vi "FPGA_LASER_4SETUP_Feb19_2016.vi"() -> ()   [LabVIEW 2015]
uses:
  <vilib>/rvi/Emulation/niFpgaGetClockAttributes.vi
  <vilib>/rvi/Emulation/niFpgaSctlEmulationGetInTimedLoop.vi
  <vilib>/rvi/Emulation/niFpgaEmulationReportErrorSimple.vi
  <vilib>/rvi/eio/common/nirviEmuTemplateMethod_errors.vi
  <vilib>/rvi/interface/RandomDataEmulation/niFpgaRandomDataHandleErrors.vi
  <vilib>/rvi/Emulation/niFpgaCriticalErrorInLSC.vi
  <vilib>/eio/EIONode/EIONode.xnode
  <vilib>/rvi/DataTransferAndStorage/Container/XNode/niFpgaContainer.xnode
  <vilib>/rvi/interface/RandomDataEmulation/nirviRandomDataFpgaReadWriteTemplate.vi
panel:
  out "Tick Count(Ticks) J5":u32 caption="Tick Count(Ticks)"
  out "Tick Count(Ticks) J8":u32 caption="Tick Count(Ticks)"
  out "Tick Count(Ticks) J4":u32 caption="Tick Count(Ticks)"
  out "Tick Count(Ticks) J1":u32 caption="Tick Count(Ticks)"
  in  "stop LED illumination J8":bool
  in  "Low Period (ticks) J8":u32=40000000
  in  "High Period (ticks) J8":u32=40000000
  in  "Apply J8":bool
  in  "Output Enable J8":bool
  in  "FPGA Stop J8":bool
  in  "Half-clock time J8":u32=10
  out "ConnectorA/DIO0 J8":bool=TRUE
  out "Frame Count J8":i16=5
  in  "IRQ Bit (0-31) J8":u8
  in  "Wait Until IRQ Cleared? J8":bool
  out "Timed Out? J8":bool
  out "ConnectorA/AI0 J8":u16=44020
  out "ConnectorA/DIO1 J8":bool
  in  "double number of samples to take per frame J8":u16=1540
  in  "Half-clocks between frames J8":u16=1600
  in  "ConnectorA/AO1 J8":u16
  in  "stop LED illumination J4":bool
  in  "Low Period (ticks) J4":u32=40000000
  in  "High Period (ticks) J4":u32=40000000
  in  "Apply J4":bool
  in  "Output Enable J4":bool
  in  "FPGA Stop J4":bool
  in  "Half-clock time J4":u32=10
  out "ConnectorB/DIO0 J4":bool=TRUE
  out "Frame Count J4":i16=5
  in  "IRQ Bit (0-31) J4":u8
  in  "Wait Until IRQ Cleared? J4":bool
  out "Timed Out? J4":bool
  out "ConnectorB/AI0 J4":u16=44020
  out "ConnectorB/DIO1 J4":bool
  in  "double number of samples to take per frame J4":u16=1540
  in  "Half-clocks between frames J4":u16=1600
  in  "ConnectorB/AO1 J4":u16
  in  "stop LED illumination J5":bool
  in  "Low Period (ticks) J5":u32=40000000
  in  "High Period (ticks) J5":u32=40000000
  in  "Apply J5":bool
  in  "Output Enable J5":bool
  in  "FPGA Stop J5":bool
  in  "Half-clock time J5":u32=10
  out "ConnectorA/DIO0 J5":bool=TRUE
  out "Frame Count J5":i16=5
  in  "IRQ Bit (0-31) J5":u8
  in  "Wait Until IRQ Cleared? J5":bool
  out "Timed Out? J5":bool
  out "ConnectorA/AI0 J5":u16=44020
  out "ConnectorA/DIO1 J5":bool
  in  "double number of samples to take per frame J5":u16=1540
  in  "Half-clocks between frames J5":u16=1600
  in  "ConnectorA/AO0 J5":u16
  in  "stop LED illumination J1":bool
  in  "Low Period (ticks) J1":u32=40000000
  in  "High Period (ticks) J1":u32=40000000
  in  "Apply J1":bool
  in  "Output Enable J1":bool
  in  "FPGA Stop J1":bool
  in  "Half-clock time J1":u32=10
  out "ConnectorB/DIO0, J1":bool=TRUE
  out "Frame Count J1":i16=5
  in  "IRQ Bit (0-31) J1":u8
  in  "Wait Until IRQ Cleared? J1":bool
  out "Timed Out? J1":bool
  out "ConnectorB/AI0 J1":u16=44020
  out "ConnectorB/DIO1 J1":bool
  in  "double number of samples to take per frame J1":u16=1540
  in  "Half-clocks between frames J1":u16=1600
  in  "ConnectorB/AO0 J1":u16
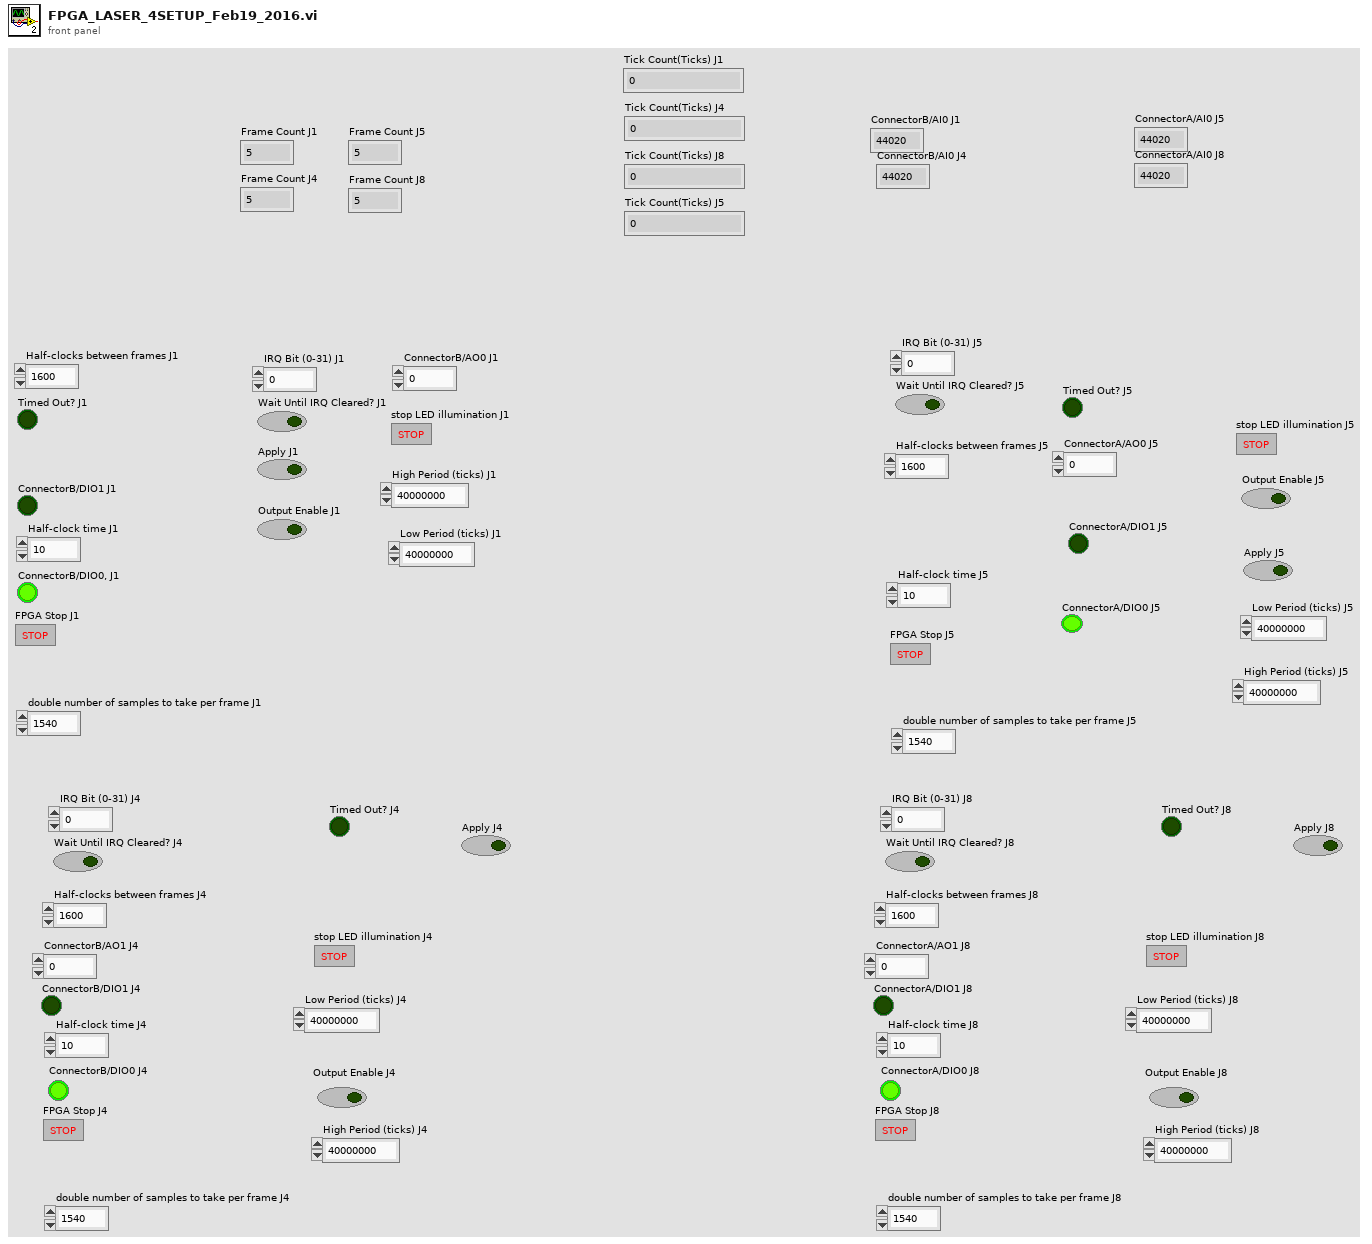
[diagram p1: front panel]
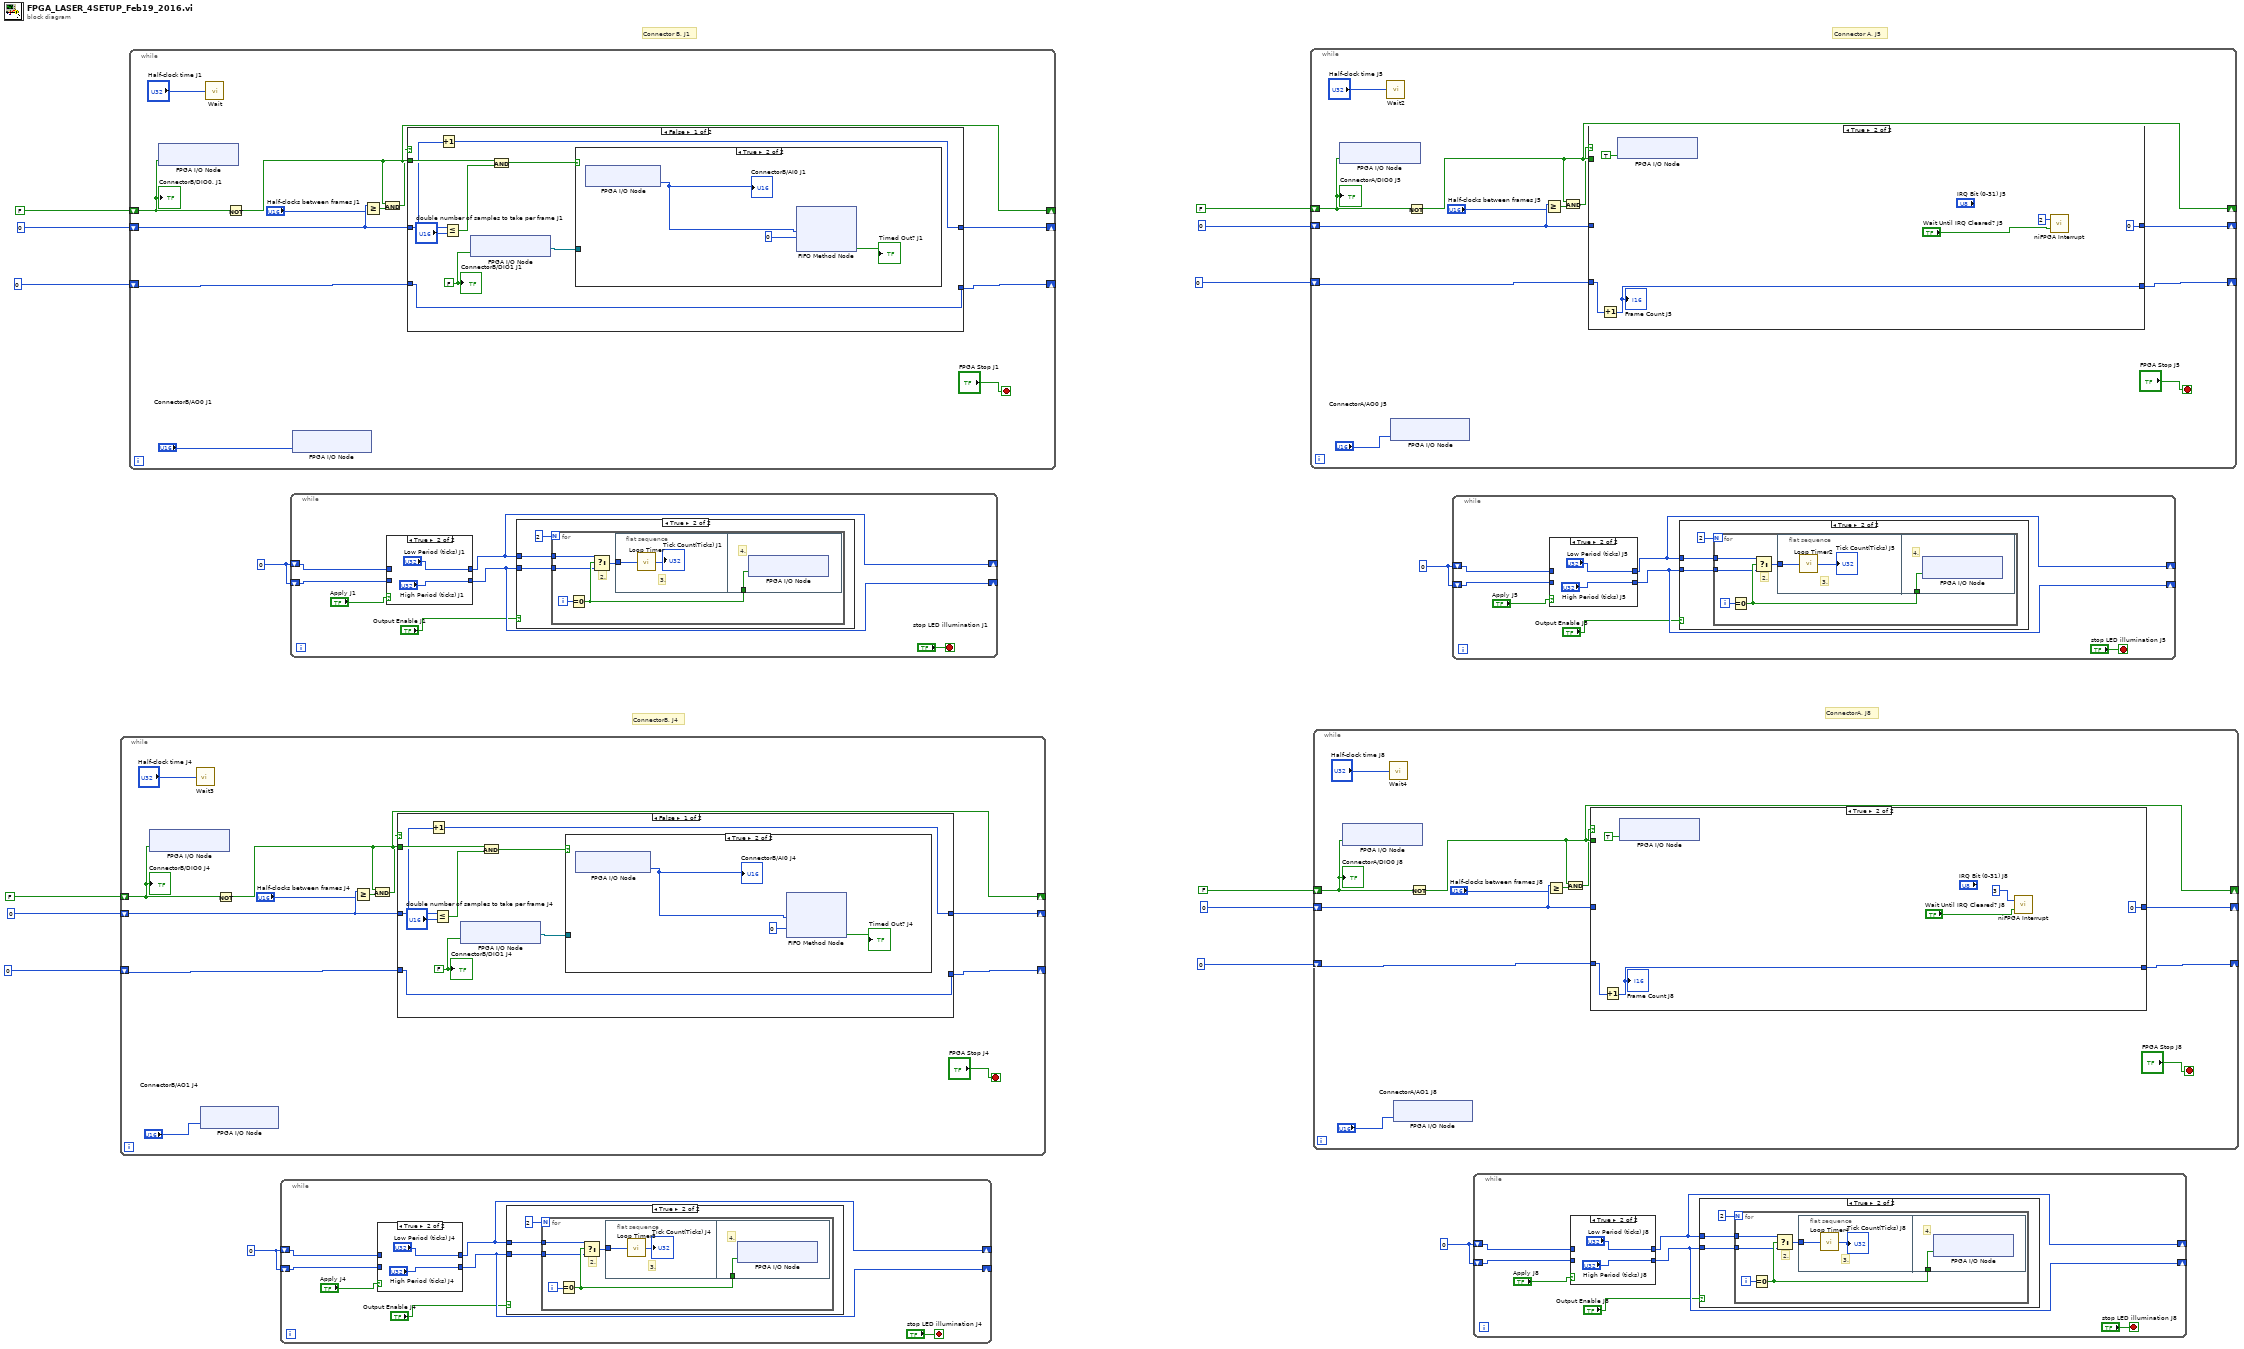
[diagram p0: block diagram]
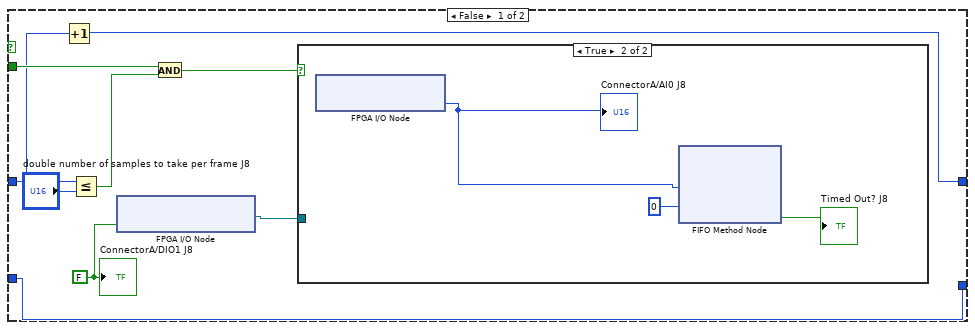
[diagram p4: hidden frame]
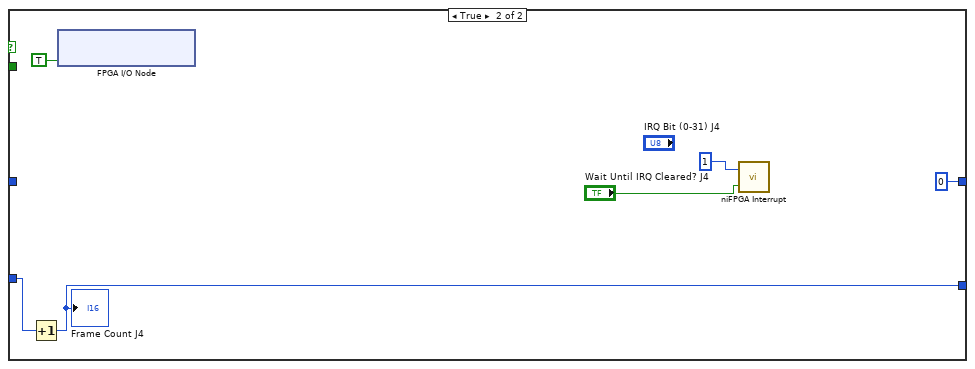
[diagram p9: hidden frame]
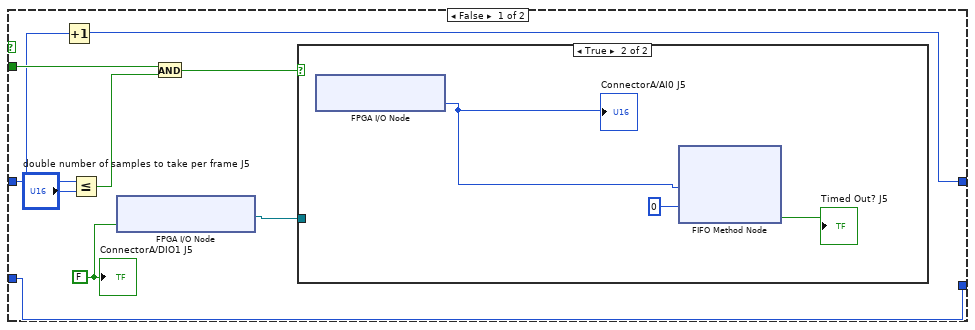
[diagram p12: hidden frame]
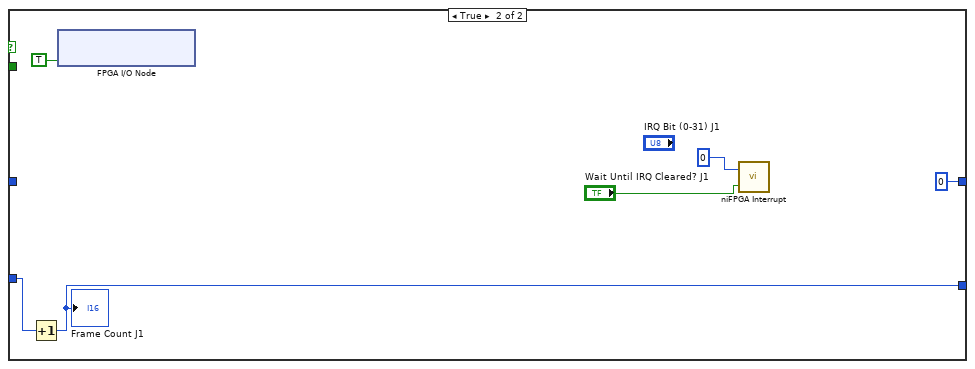
[diagram p17: hidden frame]
diagram:
  w1 = u32 0 ("High Period")
  w5 = u32 0 ("High Period")
  w9 = u32 0 ("High Period")
  w13 = u32 0 ("High Period")
  # "ConnectorA, J8"
  # "ConnectorB, J4"
  # "Connector A, J5"
  # "Connector B, J1"
  n1 = while {
    shift-right: [w27] -> _
    shift-left: FALSE ("ConnectorB/DIO0") -> [w28]
    shift-right: [w24] -> _
    shift-left: u16 0 -> [w26]
    shift-right: [w22] -> _
    shift-left: i16 0 -> [w23]
    stop <- "FPGA Stop J4" stop-if-true
    n2 = xnode "FPGA I/O Node"("ConnectorB/DIO2"=w28) -> ()  [unwired: 1 in, 1 out]
    n3 = call "Wait3"("Count(uSec)"="Half-clock time J4") -> ()  [unwired: 1 out]
    n4 = xnode "FPGA I/O Node"("ConnectorB/AO1"="ConnectorB/AO1 J4") -> ()  [unwired: 1 in, 1 out]
    n5 = Not(x=w28) -> (.not. x?=w27:bool)
    n6 = Greater Or Equal?(x=w26, y="Half-clocks between frames J4") -> (x >= y?=w20:bool)
    n7 = And(x=w27, y=w20) -> (x .and. y?=w18:bool)
    n8 = case shown="False" w18 {
      tunnel: w26 -> [w32 _]
      tunnel: [w30 u16 0] -> w24
      tunnel: w27 -> [w36 _]
      tunnel: w23 -> [w31 w44]
      tunnel: [w31 w43] -> w22
      frame False {
        w37 = FALSE ("ConnectorB/DIO1")
        n9 = Increment(x=w32) -> (x+1=w30:u16)
        n10 = Less Or Equal?(x=w32, y="double number of samples to take per frame J4") -> (x <= y?=w34:bool)
        n11 = xnode "FPGA I/O Node"("ConnectorB/DIO3"=w37) -> ("FPGA I/O Out"=w33:refnum<k21>)  [unwired: 1 in]
        n12 = And(x=w36, y=w34) -> (x .and. y?=w35:bool)
        n13 = case shown="True" w35 {
          tunnel: w33 -> [_ _]
          frame False {
          }
          frame True {
            n14 = xnode "FPGA I/O Node"() -> ("ConnectorB/AI1"=w40:u16)  [unwired: 1 in, 1 out]
            "ConnectorB/AI0 J4" <- w40
            n15 = xnode ("FIFO Method Node")("Element"=w40, "Timeout"=0) -> ("Timed Out?"=→"Timed Out? J4":bool)  [unwired: 1 in, 1 out]
          }
        }
        "ConnectorB/DIO1 J4" <- w37
      }
      frame True {
        n16 = Increment(x=w44) -> (x+1=w43:i16)
        "Frame Count J4" <- w43
        n17 = xnode "FPGA I/O Node"("ConnectorB/DIO3"=TRUE ("ConnectorB/DIO1")) -> ()  [unwired: 1 in, 1 out]
        n18 = call <vilib>:"niFPGA Interrupt.vi"("Wait Until Cleared (F)"="Wait Until IRQ Cleared? J4", "IRQ Number (0)"=u8 1) -> ()  [unwired: 1 in]
      }
    }
    "ConnectorB/DIO0 J4" <- w28
  }
  n19 = while {
    shift-right: [w57] -> _
    shift-left: FALSE ("ConnectorB/DIO0") -> [w58]
    shift-right: [w54] -> _
    shift-left: u16 0 -> [w56]
    shift-right: [w52] -> _
    shift-left: i16 0 -> [w53]
    stop <- "FPGA Stop J1" stop-if-true
    n20 = xnode "FPGA I/O Node"("ConnectorB/DIO0"=w58) -> ()  [unwired: 1 in, 1 out]
    n21 = call "Wait"("Count(uSec)"="Half-clock time J1") -> ()  [unwired: 1 out]
    n22 = Not(x=w58) -> (.not. x?=w57:bool)
    n23 = xnode "FPGA I/O Node"("ConnectorB/AO0"="ConnectorB/AO0 J1") -> ()  [unwired: 1 in, 1 out]
    n24 = Greater Or Equal?(x=w56, y="Half-clocks between frames J1") -> (x >= y?=w50:bool)
    n25 = And(x=w57, y=w50) -> (x .and. y?=w48:bool)
    n26 = case shown="False" w48 {
      tunnel: w56 -> [w62 _]
      tunnel: [w60 u16 0] -> w54
      tunnel: w57 -> [w66 _]
      tunnel: w53 -> [w61 w74]
      tunnel: [w61 w73] -> w52
      frame False {
        w67 = FALSE ("ConnectorB/DIO1")
        n27 = Increment(x=w62) -> (x+1=w60:u16)
        n28 = Less Or Equal?(x=w62, y="double number of samples to take per frame J1") -> (x <= y?=w64:bool)
        n29 = xnode "FPGA I/O Node"("ConnectorB/DIO1"=w67) -> ("FPGA I/O Out"=w63:refnum<k21>)  [unwired: 1 in]
        n30 = And(x=w66, y=w64) -> (x .and. y?=w65:bool)
        n31 = case shown="True" w65 {
          tunnel: w63 -> [_ _]
          frame False {
          }
          frame True {
            n32 = xnode "FPGA I/O Node"() -> ("ConnectorB/AI0"=w70:u16)  [unwired: 1 in, 1 out]
            "ConnectorB/AI0 J1" <- w70
            n33 = xnode ("FIFO Method Node")("Element"=w70, "Timeout"=0) -> ("Timed Out?"=→"Timed Out? J1":bool)  [unwired: 1 in, 1 out]
          }
        }
        "ConnectorB/DIO1 J1" <- w67
      }
      frame True {
        n34 = Increment(x=w74) -> (x+1=w73:i16)
        "Frame Count J1" <- w73
        n35 = xnode "FPGA I/O Node"("ConnectorB/DIO1"=TRUE) -> ()  [unwired: 1 in, 1 out]
        n36 = call <vilib>:"niFPGA Interrupt.vi"("Wait Until Cleared (F)"="Wait Until IRQ Cleared? J1", "IRQ Number (0)"=u8 0) -> ()  [unwired: 1 in]
      }
    }
    "ConnectorB/DIO0, J1" <- w58
  }
  n37 = while {
    shift-right: [w78] -> _
    shift-left: w5 -> [w82]
    shift-right: [w79] -> _
    shift-left: w5 -> [w81]
    stop <- "stop LED illumination J4" stop-if-true
    n38 = case shown="True" "Apply J4" {
      tunnel: [w96 "Low Period (ticks) J4"] -> w78
      tunnel: [w95 "High Period (ticks) J4"] -> w79
      tunnel: w82 -> [w96 _]
      tunnel: w81 -> [w95 _]
      frame False {
      }
      frame True {
      }
    }
    n39 = case shown="True" "Output Enable J4" {
      tunnel: w78 -> [_ w85]
      tunnel: w79 -> [_ w84]
      frame False {
      }
      frame True {
        n40 = for {
          N: 2 -> [_]
          tunnel: w85 -> [w88]
          tunnel: w84 -> [w87]
          i -> [w90]
          # "2."
          n41 = Equal To 0?(x=w90) -> (x = 0?=w89:bool)
          n42 = Select(t=w88, s=w89, f=w87) -> (s? t:f=w91:u32)
          n43 = flat-sequence {
            tunnel: w91 -> [w93]
            tunnel: w89 -> [w94]
            frame #0 {
              # "3."
              n44 = call "Loop Timer3"("Count(Ticks)"=w93) -> ("Tick Count(Ticks)"=→"Tick Count(Ticks) J4":u32)
            }
            frame #1 {
              # "4."
              n45 = xnode "FPGA I/O Node"("ConnectorB/DIO9"=w94) -> ()  [unwired: 1 in, 1 out]
            }
          }
        }
      }
    }
  }
  n46 = while {
    shift-right: [w100] -> _
    shift-left: w13 -> [w104]
    shift-right: [w101] -> _
    shift-left: w13 -> [w103]
    stop <- "stop LED illumination J1" stop-if-true
    n47 = case shown="True" "Apply J1" {
      tunnel: [w118 "Low Period (ticks) J1"] -> w100
      tunnel: [w117 "High Period (ticks) J1"] -> w101
      tunnel: w104 -> [w118 _]
      tunnel: w103 -> [w117 _]
      frame False {
      }
      frame True {
      }
    }
    n48 = case shown="True" "Output Enable J1" {
      tunnel: w100 -> [_ w107]
      tunnel: w101 -> [_ w106]
      frame False {
      }
      frame True {
        n49 = for {
          N: 2 -> [_]
          tunnel: w107 -> [w110]
          tunnel: w106 -> [w109]
          i -> [w112]
          # "2."
          n50 = Equal To 0?(x=w112) -> (x = 0?=w111:bool)
          n51 = Select(t=w110, s=w111, f=w109) -> (s? t:f=w113:u32)
          n52 = flat-sequence {
            tunnel: w113 -> [w115]
            tunnel: w111 -> [w116]
            frame #0 {
              # "3."
              n53 = call "Loop Timer"("Count(Ticks)"=w115) -> ("Tick Count(Ticks)"=→"Tick Count(Ticks) J1":u32)
            }
            frame #1 {
              # "4."
              n54 = xnode "FPGA I/O Node"("ConnectorB/DIO8"=w116) -> ()  [unwired: 1 in, 1 out]
            }
          }
        }
      }
    }
  }
  n55 = while {
    shift-right: [w131] -> _
    shift-left: FALSE ("ConnectorB/DIO0") -> [w132]
    shift-right: [w128] -> _
    shift-left: u16 0 -> [w130]
    shift-right: [w126] -> _
    shift-left: i16 0 -> [w127]
    stop <- "FPGA Stop J5" stop-if-true
    n56 = xnode "FPGA I/O Node"("ConnectorA/DIO0"=w132) -> ()  [unwired: 1 in, 1 out]
    n57 = call "Wait2"("Count(uSec)"="Half-clock time J5") -> ()  [unwired: 1 out]
    n58 = xnode "FPGA I/O Node"("ConnectorA/AO0"="ConnectorA/AO0 J5") -> ()  [unwired: 1 in, 1 out]
    n59 = Not(x=w132) -> (.not. x?=w131:bool)
    n60 = Greater Or Equal?(x=w130, y="Half-clocks between frames J5") -> (x >= y?=w124:bool)
    n61 = And(x=w131, y=w124) -> (x .and. y?=w122:bool)
    n62 = case shown="True" w122 {
      tunnel: w130 -> [w136 _]
      tunnel: [w134 u16 0] -> w128
      tunnel: w131 -> [w140 _]
      tunnel: w127 -> [w135 w148]
      tunnel: [w135 w147] -> w126
      frame False {
        w141 = FALSE ("ConnectorB/DIO1")
        n63 = Increment(x=w136) -> (x+1=w134:u16)
        n64 = Less Or Equal?(x=w136, y="double number of samples to take per frame J5") -> (x <= y?=w138:bool)
        n65 = xnode "FPGA I/O Node"("ConnectorA/DIO1"=w141) -> ("FPGA I/O Out"=w137:refnum<k21>)  [unwired: 1 in]
        n66 = And(x=w140, y=w138) -> (x .and. y?=w139:bool)
        n67 = case shown="True" w139 {
          tunnel: w137 -> [_ _]
          frame False {
          }
          frame True {
            n68 = xnode "FPGA I/O Node"() -> ("ConnectorA/AI0"=w144:u16)  [unwired: 1 in, 1 out]
            "ConnectorA/AI0 J5" <- w144
            n69 = xnode ("FIFO Method Node")("Element"=w144, "Timeout"=0) -> ("Timed Out?"=→"Timed Out? J5":bool)  [unwired: 1 in, 1 out]
          }
        }
        "ConnectorA/DIO1 J5" <- w141
      }
      frame True {
        n70 = Increment(x=w148) -> (x+1=w147:i16)
        "Frame Count J5" <- w147
        n71 = xnode "FPGA I/O Node"("ConnectorA/DIO1"=TRUE ("ConnectorB/DIO1")) -> ()  [unwired: 1 in, 1 out]
        n72 = call <vilib>:"niFPGA Interrupt.vi"("Wait Until Cleared (F)"="Wait Until IRQ Cleared? J5", "IRQ Number (0)"=u8 2) -> ()  [unwired: 1 in]
      }
    }
    "ConnectorA/DIO0 J5" <- w132
  }
  n73 = while {
    shift-right: [w161] -> _
    shift-left: FALSE ("ConnectorB/DIO0") -> [w162]
    shift-right: [w158] -> _
    shift-left: u16 0 -> [w160]
    shift-right: [w156] -> _
    shift-left: i16 0 -> [w157]
    stop <- "FPGA Stop J8" stop-if-true
    n74 = xnode "FPGA I/O Node"("ConnectorA/DIO2"=w162) -> ()  [unwired: 1 in, 1 out]
    n75 = call "Wait4"("Count(uSec)"="Half-clock time J8") -> ()  [unwired: 1 out]
    n76 = xnode "FPGA I/O Node"("ConnectorA/AO1"="ConnectorA/AO1 J8") -> ()  [unwired: 1 in, 1 out]
    n77 = Not(x=w162) -> (.not. x?=w161:bool)
    n78 = Greater Or Equal?(x=w160, y="Half-clocks between frames J8") -> (x >= y?=w154:bool)
    n79 = And(x=w161, y=w154) -> (x .and. y?=w152:bool)
    n80 = case shown="True" w152 {
      tunnel: w160 -> [w166 _]
      tunnel: [w164 u16 0] -> w158
      tunnel: w161 -> [w170 _]
      tunnel: w157 -> [w165 w178]
      tunnel: [w165 w177] -> w156
      frame False {
        w171 = FALSE ("ConnectorB/DIO1")
        n81 = Increment(x=w166) -> (x+1=w164:u16)
        n82 = Less Or Equal?(x=w166, y="double number of samples to take per frame J8") -> (x <= y?=w168:bool)
        n83 = xnode "FPGA I/O Node"("ConnectorA/DIO3"=w171) -> ("FPGA I/O Out"=w167:refnum<k21>)  [unwired: 1 in]
        n84 = And(x=w170, y=w168) -> (x .and. y?=w169:bool)
        n85 = case shown="True" w169 {
          tunnel: w167 -> [_ _]
          frame False {
          }
          frame True {
            n86 = xnode "FPGA I/O Node"() -> ("ConnectorA/AI1"=w174:u16)  [unwired: 1 in, 1 out]
            "ConnectorA/AI0 J8" <- w174
            n87 = xnode ("FIFO Method Node")("Element"=w174, "Timeout"=0) -> ("Timed Out?"=→"Timed Out? J8":bool)  [unwired: 1 in, 1 out]
          }
        }
        "ConnectorA/DIO1 J8" <- w171
      }
      frame True {
        n88 = Increment(x=w178) -> (x+1=w177:i16)
        "Frame Count J8" <- w177
        n89 = xnode "FPGA I/O Node"("ConnectorA/DIO3"=TRUE ("ConnectorB/DIO1")) -> ()  [unwired: 1 in, 1 out]
        n90 = call <vilib>:"niFPGA Interrupt.vi"("Wait Until Cleared (F)"="Wait Until IRQ Cleared? J8", "IRQ Number (0)"=u8 3) -> ()  [unwired: 1 in]
      }
    }
    "ConnectorA/DIO0 J8" <- w162
  }
  n91 = while {
    shift-right: [w182] -> _
    shift-left: w9 -> [w186]
    shift-right: [w183] -> _
    shift-left: w9 -> [w185]
    stop <- "stop LED illumination J5" stop-if-true
    n92 = case shown="True" "Apply J5" {
      tunnel: [w200 "Low Period (ticks) J5"] -> w182
      tunnel: [w199 "High Period (ticks) J5"] -> w183
      tunnel: w186 -> [w200 _]
      tunnel: w185 -> [w199 _]
      frame False {
      }
      frame True {
      }
    }
    n93 = case shown="True" "Output Enable J5" {
      tunnel: w182 -> [_ w189]
      tunnel: w183 -> [_ w188]
      frame False {
      }
      frame True {
        n94 = for {
          N: 2 -> [_]
          tunnel: w189 -> [w192]
          tunnel: w188 -> [w191]
          i -> [w194]
          # "2."
          n95 = Equal To 0?(x=w194) -> (x = 0?=w193:bool)
          n96 = Select(t=w192, s=w193, f=w191) -> (s? t:f=w195:u32)
          n97 = flat-sequence {
            tunnel: w195 -> [w197]
            tunnel: w193 -> [w198]
            frame #0 {
              # "3."
              n98 = call "Loop Timer2"("Count(Ticks)"=w197) -> ("Tick Count(Ticks)"=→"Tick Count(Ticks) J5":u32)
            }
            frame #1 {
              # "4."
              n99 = xnode "FPGA I/O Node"("ConnectorA/DIO8"=w198) -> ()  [unwired: 1 in, 1 out]
            }
          }
        }
      }
    }
  }
  n100 = while {
    shift-right: [w204] -> _
    shift-left: w1 -> [w208]
    shift-right: [w205] -> _
    shift-left: w1 -> [w207]
    stop <- "stop LED illumination J8" stop-if-true
    n101 = case shown="True" "Apply J8" {
      tunnel: [w222 "Low Period (ticks) J8"] -> w204
      tunnel: [w221 "High Period (ticks) J8"] -> w205
      tunnel: w208 -> [w222 _]
      tunnel: w207 -> [w221 _]
      frame False {
      }
      frame True {
      }
    }
    n102 = case shown="True" "Output Enable J8" {
      tunnel: w204 -> [_ w211]
      tunnel: w205 -> [_ w210]
      frame False {
      }
      frame True {
        n103 = for {
          N: 2 -> [_]
          tunnel: w211 -> [w214]
          tunnel: w210 -> [w213]
          i -> [w216]
          # "2."
          n104 = Equal To 0?(x=w216) -> (x = 0?=w215:bool)
          n105 = Select(t=w214, s=w215, f=w213) -> (s? t:f=w217:u32)
          n106 = flat-sequence {
            tunnel: w217 -> [w219]
            tunnel: w215 -> [w220]
            frame #0 {
              # "3."
              n107 = call "Loop Timer4"("Count(Ticks)"=w219) -> ("Tick Count(Ticks)"=→"Tick Count(Ticks) J8":u32)
            }
            frame #1 {
              # "4."
              n108 = xnode "FPGA I/O Node"("ConnectorA/DIO9"=w220) -> ()  [unwired: 1 in, 1 out]
            }
          }
        }
      }
    }
  }
